vi "CAN Reset.vi"(8 "error in (no error)":errorcluster, 11 "Channel":u16) -> (0 "error out":errorcluster, 3 "function return":u32)   [LabVIEW 2017, in "PCANBasic_eX.lvlib"]
doc: "TPCANStatus __stdcall CAN_Reset(\n TPCANHandle Channel);"
uses:
  PCANBasic_eX.lvlib
  PCANBasic.dll
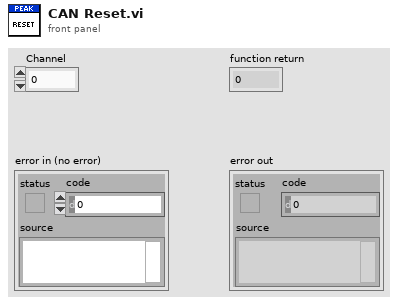
[diagram p1: front panel]
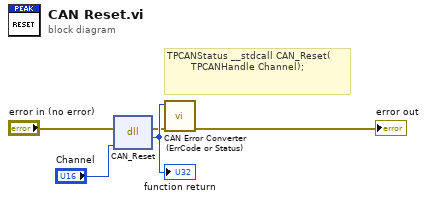
[diagram p0: block diagram]
diagram:
  # "TPCANStatus __stdcall CAN_Reset(\n        TPCANHandle Channel);"
  n1 = dll-call lib="PCANBasic.*" fn="CAN_Reset"(error in="error in (no error)", "Channel"="Channel") -> (error out=w2:errorcluster, w5:u32)  [unwired: 3 in, 1 out]
  "function return" <- w5
  n2 = call "CAN Error Converter (ErrCode or Status).vi"("error in (no error)"=w2, "error code"=w5) -> ("error out"=→"error out":errorcluster)  [unwired: 9 in]
